vi "Discovery Service - Find Service.vi"(0 "discovery address":string="localhost:42000", 5 "Measurement Name":string, 7 "Measurement Service":string, 11 "error in":errorcluster) -> (4 "Cancelled?":bool, 6 "Measurement location":string, 8 "Measurement port":string, 15 "error out":errorcluster)   [LabVIEW 2020, in "InstrumentStudioPlugin_RenameMe.lvlib"]
uses:
  InstrumentStudioPlugin_RenameMe.lvlib
  <vilib>/TAF/Discovery Client/RPC Messages/NIMeasurementServices_EnumerateServicesRequest.ctl
  <vilib>/TAF/Discovery Client/RPC Messages/NIMeasurementServices_ResolveServiceRequest.ctl
  a01f274c-073a-4d5b-a5b9-6f5bc39487d5.vi
  <vilib>/Comparison/Equal/Equal Functor/Equal Functor.lvclass
  <vilib>/TAF/Discovery Client/Discovery_client.lvlib
panel:
  in  "Measurement Service":i32(listbox)
  in  "Measurement Service Class":i32(listbox)
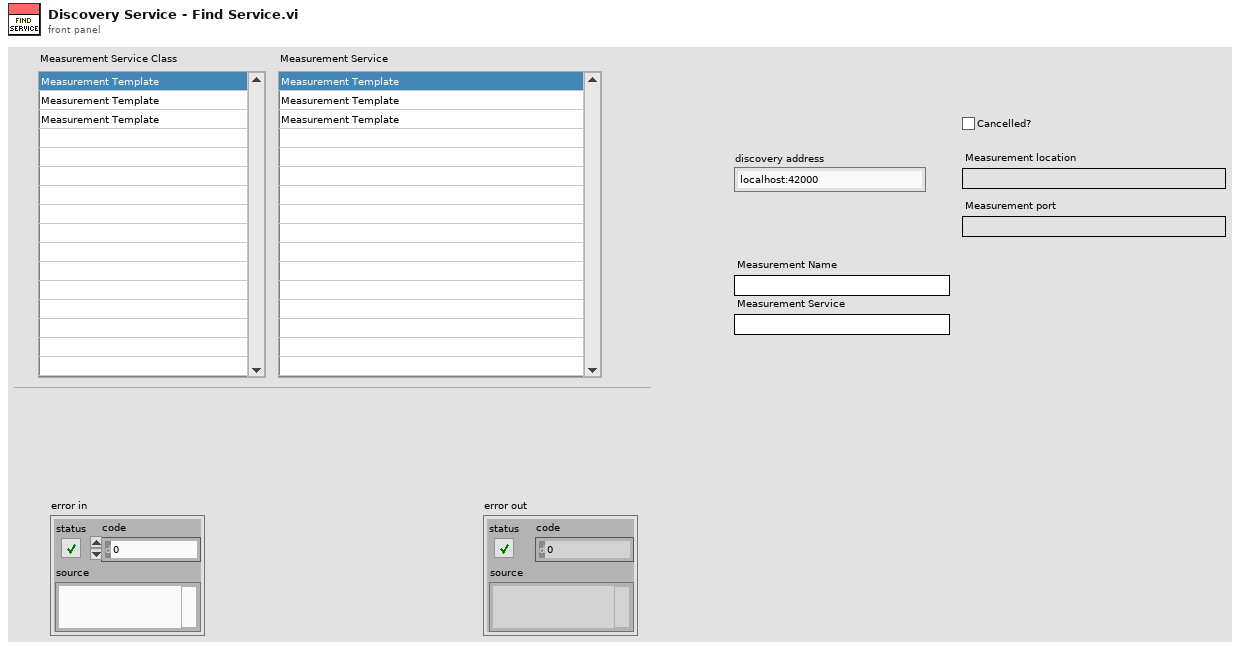
[diagram p1: front panel]
types:
  T1 = typedef "Discovery_client.lvlib/NIMeasurementServices_EnumerateServicesRequest.ctl" = cluster{"required_service":string}
  T2 = typedef "gprc-lvsupport-release.lvlib/grpcId.ctl" = u64
  T3 = typedef "Discovery_client.lvlib/NIMeasurementServices_EnumerateServicesResponse.ctl" = cluster{"available_services":T4[]}
  T4 = typedef "Discovery_client.lvlib/NIMeasurementServices_ServiceDescriptor.ctl" = cluster{"service_id":string, "name":string, "description_url":string, "service_class":string}
  T5 = typedef "Discovery_client.lvlib/NIMeasurementServices_ResolveServiceRequest.ctl" = cluster{"request_data_location":string, "required_service_class":string}
  T6 = typedef "Discovery_client.lvlib/NIMeasurementServices_ServiceLocation.ctl" = cluster{"location":string, "optimal_route":string, "insecure_port":string, "ssl_authenticated_port":string}
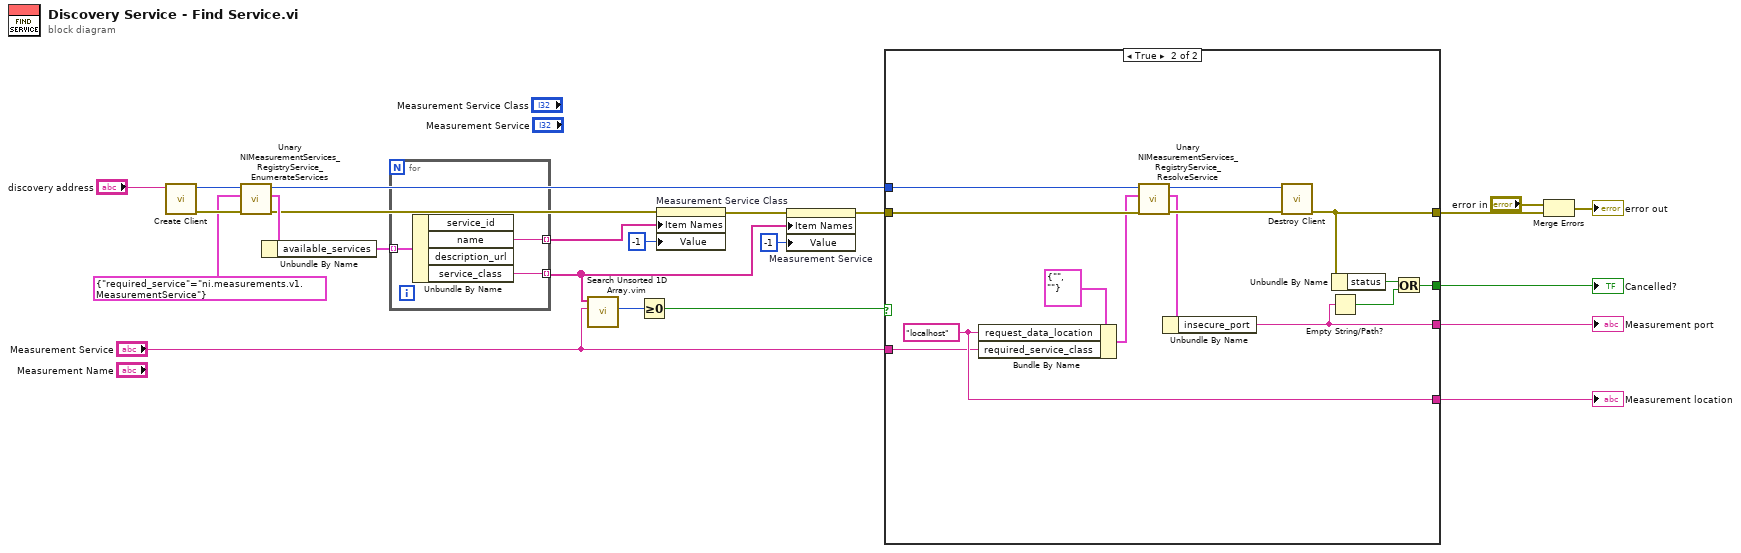
[diagram p0: block diagram]
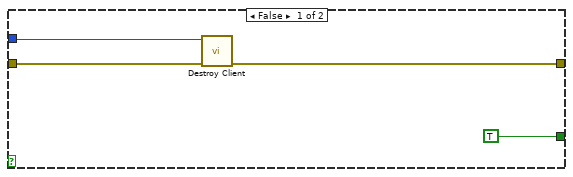
[diagram p2: hidden frame]
diagram:
  n1 = call <vilib>:"Create Client.vi"("address"="discovery address") -> ("error out"=w19:errorcluster, "gRPC ID Out"=w21:T2)  [unwired: 9 in]
  n2 = call <vilib>:"Unary NIMeasurementServices_RegistryService_EnumerateServices.vi"("error in"=w19, "Request Data"=T1 {"required_service"="ni.measurements.v1.MeasurementService"}, "gRPC ID"=w21) -> ("error out"=w16:errorcluster, "Response Data"=w18:T3, "gRPC ID out"=w20:T2)  [unwired: 6 in]
  n3 = Unbundle By Name(w18) -> ("available_services"=w17:T4[])
  n4 = for {
    tunnel: w17 -> [w26] mode=indexing
    tunnel: [w25] -> w12 mode=indexing
    tunnel: [w24] -> w7 mode=indexing
    n5 = Unbundle By Name(w26) -> ("name"=w25:string, "service_class"=w24:string)  [unwired: 2 out]
  }
  n6 = call "Search Unsorted 1D Array.vim"("element"="Measurement Service", "unsorted 1D array"=w7) -> ("index of element"=w5:i32)  [unwired: 9 in]
  n7 = Greater Or Equal To 0?(x=w5) -> (x >= 0?=w4:bool)
  n8 = property on="Measurement Service Class" class="LstBox (strict)"(error in=w16, "Item Names"=w12, "Value"=-1 ("Available Measurement Service")) -> (error out=w14:errorcluster)  [unwired: 1 in, 1 out]
  n9 = property on="Measurement Service" class="LstBox (strict)"(error in=w14, "Item Names"=w7, "Value"=-1 ("Measurement Service")) -> (error out=w13:errorcluster)  [unwired: 1 in, 1 out]
  n10 = case shown="True" w4 {
    tunnel: [_ w44] -> w23
    tunnel: w20 -> [w27 w41]
    tunnel: w13 -> [w29 w40]
    tunnel: [w28 w32] -> w10
    tunnel: [_ w37] -> w9
    tunnel: [TRUE w36] -> w8
    tunnel: "Measurement Service" -> [_ w33]
    frame False {
      n11 = call <vilib>:"Destroy Client.vi"("error in"=w29, "gRPC ID"=w27) -> ("error out"=w28:errorcluster)  [unwired: 9 in]
    }
    frame True {
      w44 = "localhost" ("request_data_location")
      n12 = Bundle By Name(cluster=T5 {"request_data_location"="", "required_service_class"=""} ("Request Data"), "request_data_location"=w44, "required_service_class"=w33) -> (w39:T5)
      n13 = call <vilib>:"Unary NIMeasurementServices_RegistryService_ResolveService.vi"("error in"=w40, "Request Data"=w39, "gRPC ID"=w41) -> ("error out"=w43:errorcluster, "Response Data"=w38:T6, "gRPC ID out"=w42:T2)  [unwired: 6 in]
      n14 = Unbundle By Name(w38) -> ("insecure_port"=w37:string)
      n15 = call <vilib>:"Destroy Client.vi"("error in"=w43, "gRPC ID"=w42) -> ("error out"=w32:errorcluster)  [unwired: 9 in]
      n16 = Empty String/Path?(string/path=w37) -> (empty?=w34:bool)
      n17 = Unbundle By Name(w32) -> ("status"=w35:bool)
      n18 = Or(x=w35, y=w34) -> (x .or. y?=w36:bool)
    }
  }
  "Cancelled?" <- w8
  "Measurement location" <- w23
  "Measurement port" <- w9
  n19 = Merge Errors("error in", w10) -> (→"error out":errorcluster)
